vi "globalRefs_rigDependent.vi"() -> ()   [LabVIEW 2015]
uses:
  X:/Lab/Labmembers/Shane Nichols/Labview/InstrumentControl20190423/general_utilities.llb/multiDeviceSynchronization.ctl
panel:
  in  "inputChannelRefs":T1={"PMTA"={"name"="PMT1", "physicalChannel"="Dev3/ai0", "Active?"=TRUE}, "PMTB"={"name"="PMT2", "physicalChannel"="Dev3/ai1", "Active?"=TRUE}, "cameraExposureOut"={"name"="PMT2", "physicalChannel"="Dev3/ai1", "Active?"=TRUE}, "galvoPosX"={"name"="PMT1", "physicalChannel"="Dev3/ai0", "Active?"=TRUE}, "galvoPosY"={"name"="PMT1", "physicalChannel"="Dev3/ai0", "Active?"=TRUE}, "blackflyCounter"={"name"="PMT1", "physicalChannel"="Dev3/ai0", "Active?"=TRUE}}
  in  "outputChannelRefs":T2={"galvoX"={"name"="galvoX", "physicalChannel"="Dev3/ao0"}, "galvoY"={"name"="galvoY", "physicalChannel"="Dev3/ao1"}, "mod488"={"name"="mod488", "physicalChannel"="Dev3/ao2"}, "modTiSaph"={"name"="modTiSaph", "physicalChannel"="Dev3/ao3"}, "shutter488"={"name"="shutter488", "physicalChannel"="Dev3/port0/line3"}, "shutterTiSaph"={"name"="shutterTiSaph", "physicalChannel"="Dev3/port0/line1"}, " shutter635"={"name"="shutter635", "physicalChannel"="Dev3/port0/line2"}, " shutter635-2"={"name"="shutter635", "physicalChannel"="Dev3/port0/line2"}, "triggerCamera"={"name"="cameraTrigger", "physicalChannel"="Dev3/port0/line0"}, "triggerBlackfly"={"name"="cameraTrigger", "physicalChannel"="Dev3/port0/line0"}}
  in  "clockSourcePresents":T3(array[cluster])
  in  "daqTrigger":T4={"Type"=0, "source"="/Dev1/PFI15", "equivalentChannel"=""} {"Type" items=["No Trigger", "Digital Start"]}
  in  "multiDeviceSynchronization":T5[](array[typedef])
  in  "rigName":string="AdaptiveUpright"
  # "Hard Coded Port References. These are compile time settings that are rig dependent. They configure the DAQ mostly"
  # "*use the port map in NI MAX to figure out what channel corresponsds to the trigger terminal (Source)."
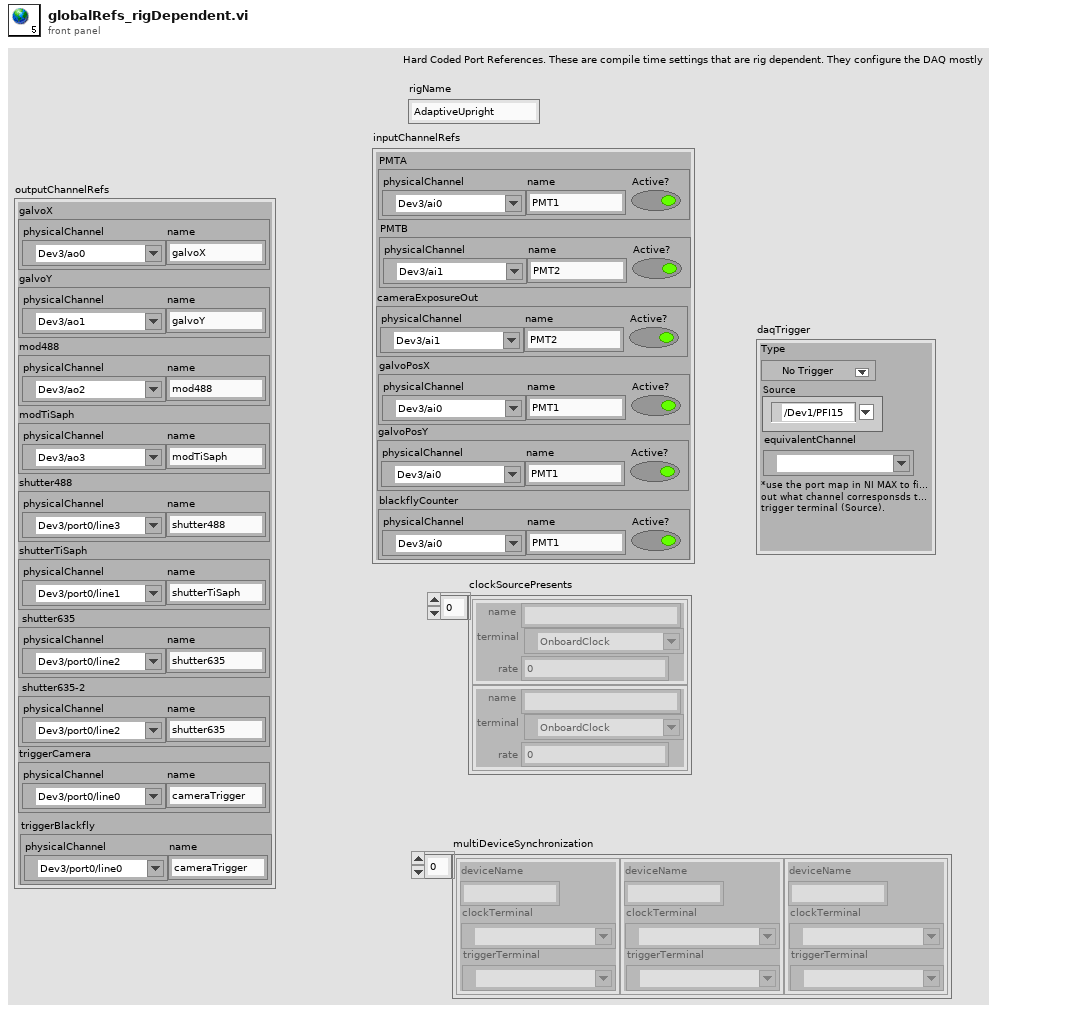
[diagram p1: front panel]
types:
  T1 = cluster{"PMTA":cluster{"name":string, "physicalChannel":tag, "Active?":bool}, "PMTB":cluster{"name":string, "physicalChannel":tag, "Active?":bool}, "cameraExposureOut":cluster{"name":string, "physicalChannel":tag, "Active?":bool}, "galvoPosX":cluster{"name":string, "physicalChannel":tag, "Active?":bool}, "galvoPosY":cluster{"name":string, "physicalChannel":tag, "Active?":bool}, "blackflyCounter":cluster{"name":string, "physicalChannel":tag, "Active?":bool}}
  T2 = cluster{"galvoX":cluster{"name":string, "physicalChannel":tag}, "galvoY":cluster{"name":string, "physicalChannel":tag}, "mod488":cluster{"name":string, "physicalChannel":tag}, "modTiSaph":cluster{"name":string, "physicalChannel":tag}, "shutter488":cluster{"name":string, "physicalChannel":tag}, "shutterTiSaph":cluster{"name":string, "physicalChannel":tag}, " shutter635":cluster{"name":string, "physicalChannel":tag}, " shutter635-2":cluster{"name":string, "physicalChannel":tag}, "triggerCamera":cluster{"name":string, "physicalChannel":tag}, "triggerBlackfly":cluster{"name":string, "physicalChannel":tag}}
  T3 = cluster{"name":string, "terminal":tag, "rate":dbl}[]
  T4 = cluster{"Type":u16, "source":tag, "equivalentChannel":tag}
  T5 = typedef "multiDeviceSynchronization.ctl" = cluster{"clockTerminal":tag, "triggerTerminal":tag, "deviceName":string}
diagram:
